vi "FisherPaykel Initialize.vi"(7 "Debug":bool, 8 "Error In":errorcluster, 11 "VISA Refnum in":refnum<visa-resource-name>) -> (0 "Error Out":errorcluster, 3 "VISA Refnum out":refnum<visa-resource-name>)   [LabVIEW 2016]
uses:
  Type Definitions/Fisher Paykel Main Command.ctl
  Type Definitions/Checksum.ctl
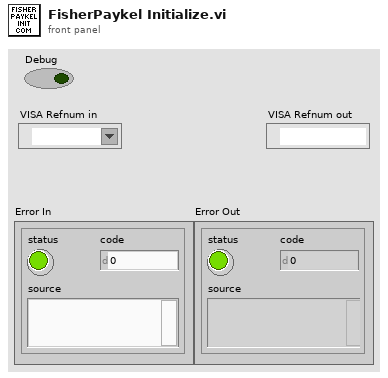
[diagram p1: front panel]
types:
  T1 = typedef "Fisher Paykel Main Command.ctl" = string
  T2 = typedef "Checksum.ctl" = string
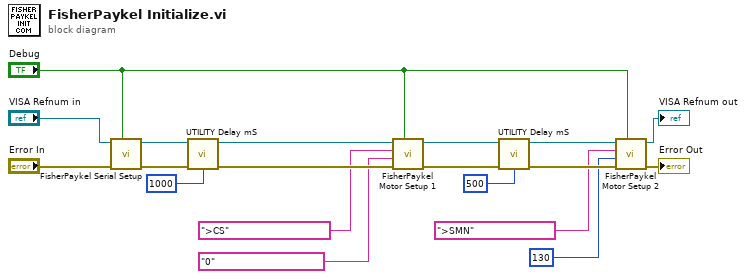
[diagram p0: block diagram]
diagram:
  n1 = call "FisherPaykel Serial Setup.vi"("Debug"="Debug", "error in (no error)"="Error In", "VISA Refnum in"="VISA Refnum in") -> ("Error Out"=w9:errorcluster, "VISA Refnum out"=w11:refnum<visa-resource-name>)  [unwired: 7 in]
  n2 = call "UTILITY Delay mS.vi"("Error In"=w9, "milliseconds to wait"=u32 1000) -> ("Error Out"=w8:errorcluster)  [unwired: 13 in]
  n3 = call "FisherPaykel Motor Setup 1.vi"("Debug"="Debug", "error in (no error)"=w8, "Command Modifier"=T2 "0", "Main Command"=T1 ">CS", "VISA Refnum in"=w11) -> ("error out"=w6:errorcluster, "VISA Refnum out"=w12:refnum<visa-resource-name>)  [unwired: 5 in]
  n4 = call "UTILITY Delay mS.vi"("Error In"=w6, "milliseconds to wait"=u32 500) -> ("Error Out"=w5:errorcluster)  [unwired: 13 in]
  n5 = call "FisherPaykel Motor Setup 2.vi"("Debug"="Debug", "Error In"=w5, "Motor Number"=u16 130, "Main Command"=T1 ">SMN", "VISA Refnum in"=w12) -> ("Error Out"=→"Error Out":errorcluster, "VISA Refnum out"=→"VISA Refnum out":refnum<visa-resource-name>)  [unwired: 5 in]
